vi "SendClusterError(SubVI).vi"(8 "error in (no error)":errorcluster, 11 "Cluster in":refnum<vi>) -> (0 "error out":errorcluster)   [LabVIEW 2018]
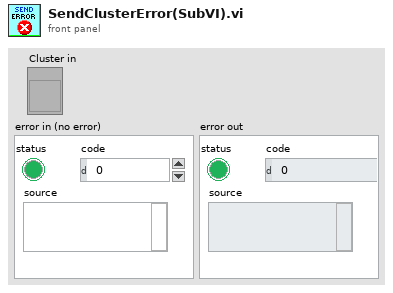
[diagram p1: front panel]
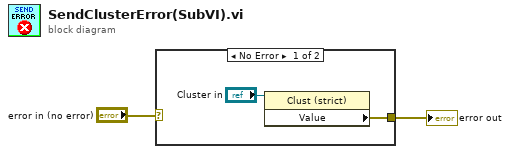
[diagram p0: block diagram]
diagram:
  n1 = case shown="No Error" "error in (no error)" {
    selector: "error in (no error)" -> [_ w5]
    tunnel: [w3 w5] -> w2
    frame No Error {
      n2 = property on="Property Node" class="Clust (strict)"(reference="Cluster in") -> ("Value"=w3:errorcluster)  [unwired: 1 in, 2 out]
    }
    frame Error {
    }
  }
  "error out" <- w2
